vi "Test.vi"(0 "Traverse Algorithm in":refnum<class "Format Into String.lvclass">, 5 "Terminal To Identify":refnum<vi>, 11 "error in (no error)":errorcluster) -> (4 "Traverse Algorithm out":refnum<class "Format Into String.lvclass">, 6 "Terminal for Traversal Continuation":refnum<vi>[](array[refnum]), 8 "Node Identified":bool, 15 "error out":errorcluster)   [LabVIEW 2019, in "MVA Message Mapper.lvlib" / "Format Into String.lvclass"]
uses:
  Format Into String.lvclass
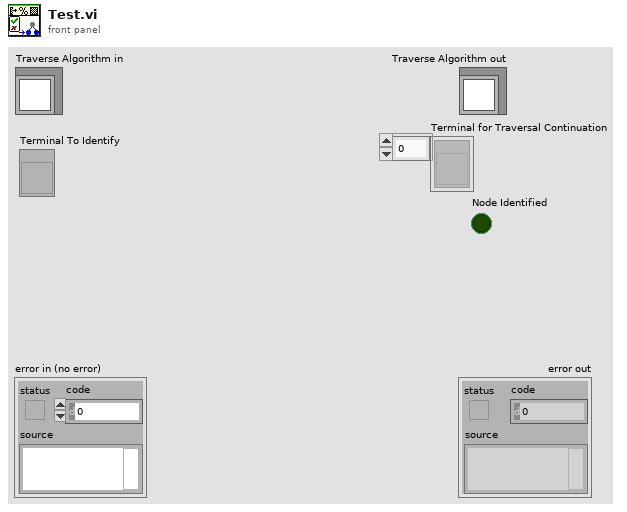
[diagram p1: front panel]
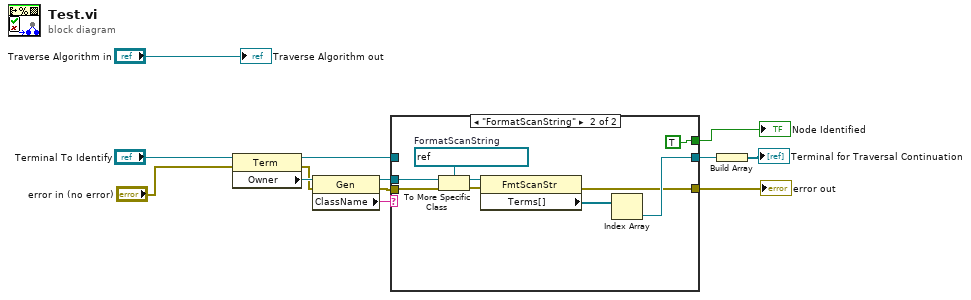
[diagram p0: block diagram]
diagram:
  n1 = property on="Property Node" class="Term"(reference="Terminal To Identify", error in="error in (no error)") -> (reference out=w9:refnum<vi>, error out=w3:errorcluster, "Owner"=w11:refnum<vi>)
  n2 = property on="Property Node" class="Gen"(reference=w11, error in=w3) -> (reference out=w5:refnum<vi>, error out=w2:errorcluster, "ClassName"=w10:string)
  n3 = case shown="\"FormatScanString\"" w10 {
    tunnel: w9 -> [w15 _]
    tunnel: [w15 w19] -> w8
    tunnel: [_ TRUE ("Node Identified")] -> w7
    tunnel: w5 -> [_ w23]
    tunnel: w2 -> [w14 w18]
    tunnel: [w14 w16] -> w1
    frame "False", Default {
    }
    frame "FormatScanString" {
      w22 = refnum<vi> refnum  # FormatScanString
      n4 = To More Specific Class(target class=w22, reference=w23, error in=w18) -> (specific class reference=w21:refnum<vi>, error out=w17:errorcluster)
      n5 = property class="FmtScanStr"(reference=w21, error in=w17) -> (error out=w16:errorcluster, "Terms[]"=w20:refnum<vi>[])  [unwired: 1 out]
      n6 = Index Array(array=w20) -> (element=w19:refnum<vi>)  [unwired: 1 in]
    }
  }
  "error out" <- w1
  "Node Identified" <- w7
  n7 = Build Array(w8) -> (→"Terminal for Traversal Continuation":refnum<vi>[])
  "Traverse Algorithm out" <- "Traverse Algorithm in"
